vi "FT10_Config Remove Comment.vi"(10 "Value In":string) -> (2 "Value without Comment":string)   [LabVIEW 2015]
doc: "Removes whitespace and everything after \"#\" sign which marks comments"
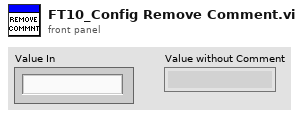
[diagram p1: front panel]
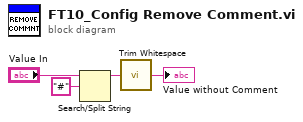
[diagram p0: block diagram]
diagram:
  n1 = Search/Split String(string="Value In", search string/char (-)="#") -> (substring before match=w2:string)  [unwired: 1 in, 2 out]
  n2 = call <vilib>:"Trim Whitespace.vi"("string"=w2) -> ("trimmed string"=→"Value without Comment":string)  [unwired: 1 in]
